vi "Get Topology from JSON.vi"(8 "error in (no error)":errorcluster, 11 "Capabilities JSON In":string) -> (0 "error out":errorcluster, 2 "JSON Tree Passthrough (JSON Array)":variant, 3 "Array Size":i32)   [LabVIEW 2015, in "SLSC Switch.lvlib" / "SLSC Switch.lvclass"]
uses:
  SLSC Switch.lvclass
  <vilib>/LVH/i3 JSON/JSON Parsing/Get Object Parameter Files/Get Object Parameter - Array.vi
  <vilib>/LVH/i3 JSON/i3-json.lvlib
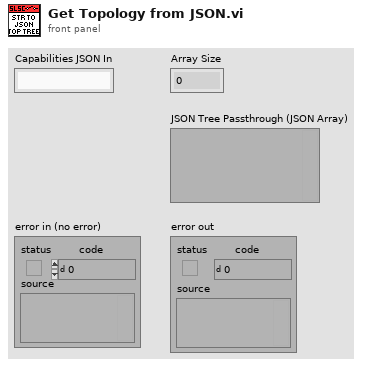
[diagram p1: front panel]
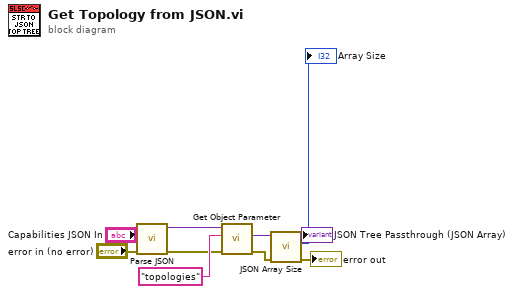
[diagram p0: block diagram]
diagram:
  n1 = call <vilib>:"Parse JSON.vi"("error in (no error)"="error in (no error)", "JSON String"="Capabilities JSON In") -> ("error out"=w4:errorcluster, "JSON Tree"=w6:variant)  [unwired: 6 in, 2 out]
  n2 = call-poly <vilib>:"Get Object Parameter.vi"("error in (no error)"=w4, "Parameter Name"="topologies", "JSON Tree In (JSON Object)"=w6) -> ("error out"=w3:errorcluster, "JSON Array"=w8:variant)  [unwired: 5 in, 2 out]
  n3 = call <vilib>:"JSON Array Size.vi"("error in (no error)"=w3, "JSON Tree In (JSON Array)"=w8) -> ("error out"=→"error out":errorcluster, "Array Size"=→"Array Size":i32, "JSON Tree Passthrough (JSON Array)"=→"JSON Tree Passthrough (JSON Array)":variant)  [unwired: 7 in]
